vi "PCO_SetPixelRate.vi"(8 "error in (no error)":errorcluster {"code" format="%x"}, 10 "dwPixelRate":u32, 11 "ph":u64) -> (0 "error out":errorcluster {"code" format="%x"}, 2 "ErrorMessage":i32 format="%x", 3 "ph out":u64)   [LabVIEW 2019, in "SDK.lvlib" / "ImageSensor.lvlib"]
doc: "<b>Description:</b>\nThis function does set the pixel rate for the sensor readout. Only values, which are listed in the parameter list dwPixelRateDESC of the PCO_Description structure, are accepted.\nFor pco.edge 5.5 with Camera Link interface PCO_SetTransferParameter and PCO_SetActiveLookuptable with appropriate parameters must be called. See chapter IMAGE AREA SELECTION (ROI).\nInvalid values result in a failure response message.\nThe command will be rejected, if Recording State is [run], see PCO_GetRecordingState.\n\n<b>Supported camera type:</b>\nAll cameras\n\n<b>Descriptor dependency:</b>\nNone"
uses:
  ImageSensor.lvlib
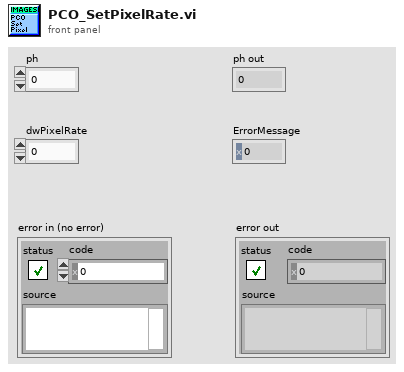
[diagram p1: front panel]
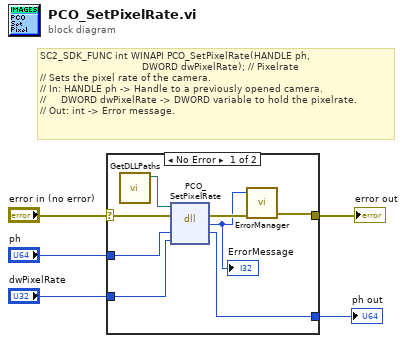
[diagram p0: block diagram]
diagram:
  # "SC2_SDK_FUNC int WINAPI PCO_SetPixelRate(HANDLE ph,\n                                  DWORD dwPixelRate); // Pixelrate\n// Sets the pixel rate of the camera.\n// In: HANDLE ph -> Handle to a previously opened camera.\n//     DWORD dwPixelRate -> DWORD variable to hold the pixelrate.\n// Out: int -> Error message."
  n1 = case shown="No Error" "error in (no error)" {
    selector: "error in (no error)" -> [w10 w15]
    tunnel: "ph" -> [w13 w14]
    tunnel: [w12 w14] -> w4
    tunnel: "dwPixelRate" -> [w11 _]
    tunnel: [w8 w15] -> w2
    frame No Error {
      n2 = call "GetDLLPaths.vi"() -> ("SC2_Cam_Path"=w6:path)  [unwired: 9 in, 2 out]
      n3 = dll-call lib="?" fn="PCO_SetPixelRate"(path in=w6, error in=w10, "ph"=w13, "dwPixelRate"=w11) -> (error out=w9:errorcluster, "return type"=w7:i32, "ph"=w12:u64)  [unwired: 2 in, 1 out]
      "ErrorMessage" <- w7
      n4 = call "ErrorManager.vi"("error in (no error)"=w9, "error code"=w7) -> ("error out"=w8:errorcluster)  [unwired: 3 in]
    }
    frame Error {
    }
  }
  "ph out" <- w4
  "error out" <- w2
